vi "Untitled 1.vi"() -> ()   [LabVIEW 2017]
uses:
  <vilib>/Platform/TimedLoop/XDataNode/timing_clust.ctl
  <vilib>/Platform/TimedLoop/XDataNode/nitl_modes.ctl
  <vilib>/Platform/TimedLoop/XDataNode/wakeup.ctl
  <vilib>/platform/TimedLoop/XDataNode/XDataNode.xnode
  <vilib>/Platform/TimedLoop/XDataNode/XDNodeRunTimeDep.lvlib
panel:
  in  "Initialize integral 2":bool
  out "Analog2":dbl(knob) scale=0.0..5.0
  out "Waveform Chart 2":cluster{"Ref2":dbl, dbl}(graph)
  out "Pos2":dbl(knob) scale=0.0..360.0
  in  "Ref2":dbl(slide) scale=-720.0..720.0
  in  "stop":bool
  in  "Kd":dbl(slide) scale=0.0..10.0
  in  "Ki":dbl(slide) scale=0.0..10.0
  in  "Kp":dbl(slide) scale=0.0..10.0
  out "Analog1":dbl(knob) scale=0.0..5.0
  out "Waveform Chart":cluster{"Ref 1":dbl, dbl}(graph)
  in  "Initialize integral 1":bool
  in  "Ref 1":dbl(slide) scale=-720.0..720.0
  out "Pos 1":dbl(knob) scale=0.0..360.0
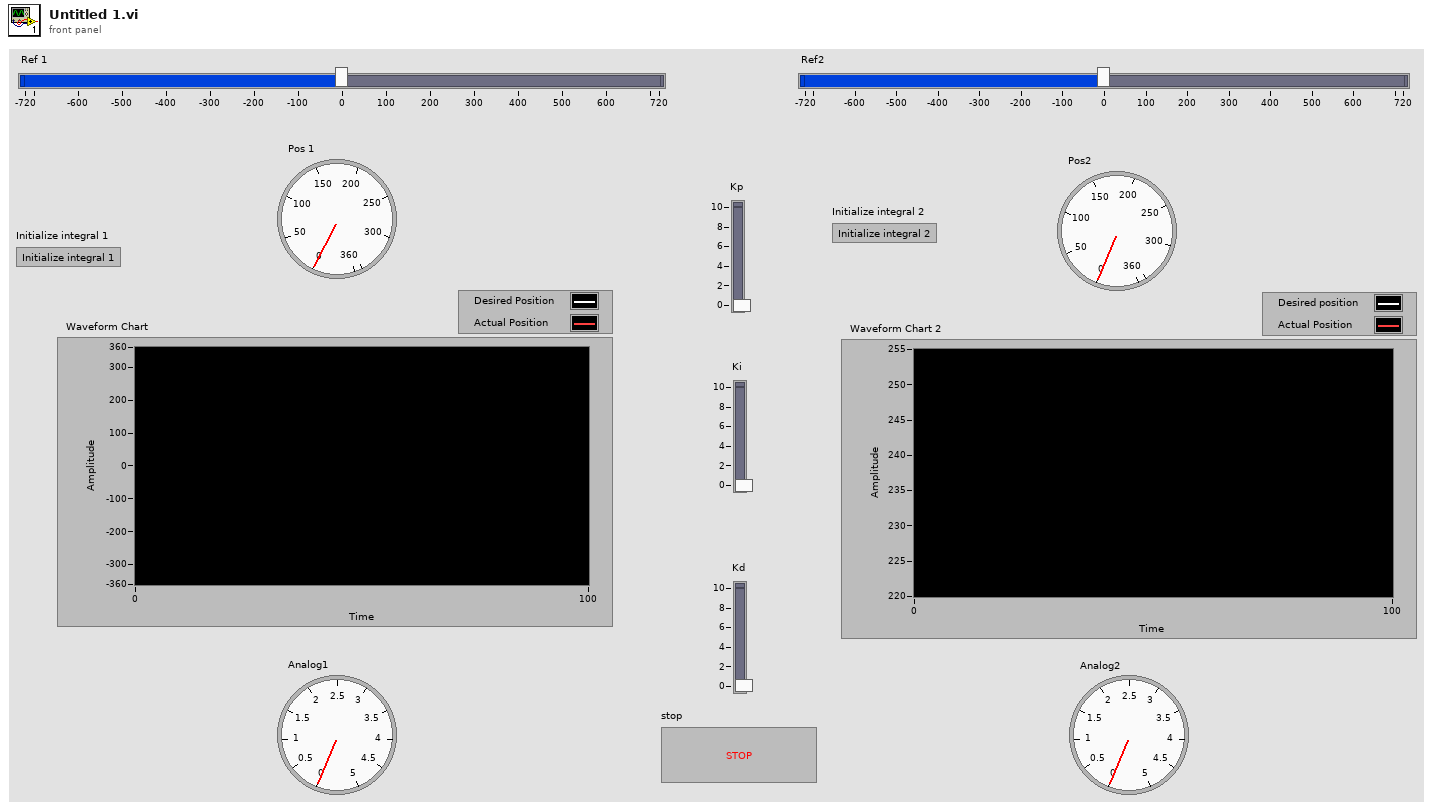
[diagram p1: front panel]
types:
  T1 = typedef "XDNodeRunTimeDep.lvlib/timing_clust.ctl" = cluster{"Expected End [f-1]":u64, "Actual End [f-1]":u64, "Finished Late? [f-1]":bool, "Expected End [i-1]":u64, "Actual End [i-1]":u64, "Finished Late? [i-1]":bool, "Expected Start [i]":u64, "Actual Start [i]":u64, "Expected Start [f]":u64, "Actual Start [f]":u64, "Source Name":string, "Structure Name":string, "Period":i64, "Deadline":i64, "Offset":i64, "Start":i64, "Priority":i32, "Timeout":i32, "Mode":T2, "Wakeup Reason":T3, "Error":errorcluster, "Source Type":string, "Secondary Source Type":string, "Global End Time":u64, "Global Start Time":u64, "Frame Duration":u64, "Iteration Duration":u64, "Assigned CPU":i32, "I/O Scan Engine Mode":u32}
  T2 = typedef "XDNodeRunTimeDep.lvlib/nitl_modes.ctl" = enum32{"No Change", "Process missed periods, maintain original phase", "Discard missed periods, maintain original phase", "Process missed periods, ignore original phase", "Discard missed periods, ignore original phase"}
  T3 = typedef "XDNodeRunTimeDep.lvlib/wakeup.ctl" = enum32{"Normal", "Aborted", "Asynchronous wakeup", "Timing source error", "Timed loop error", "Timeout"}
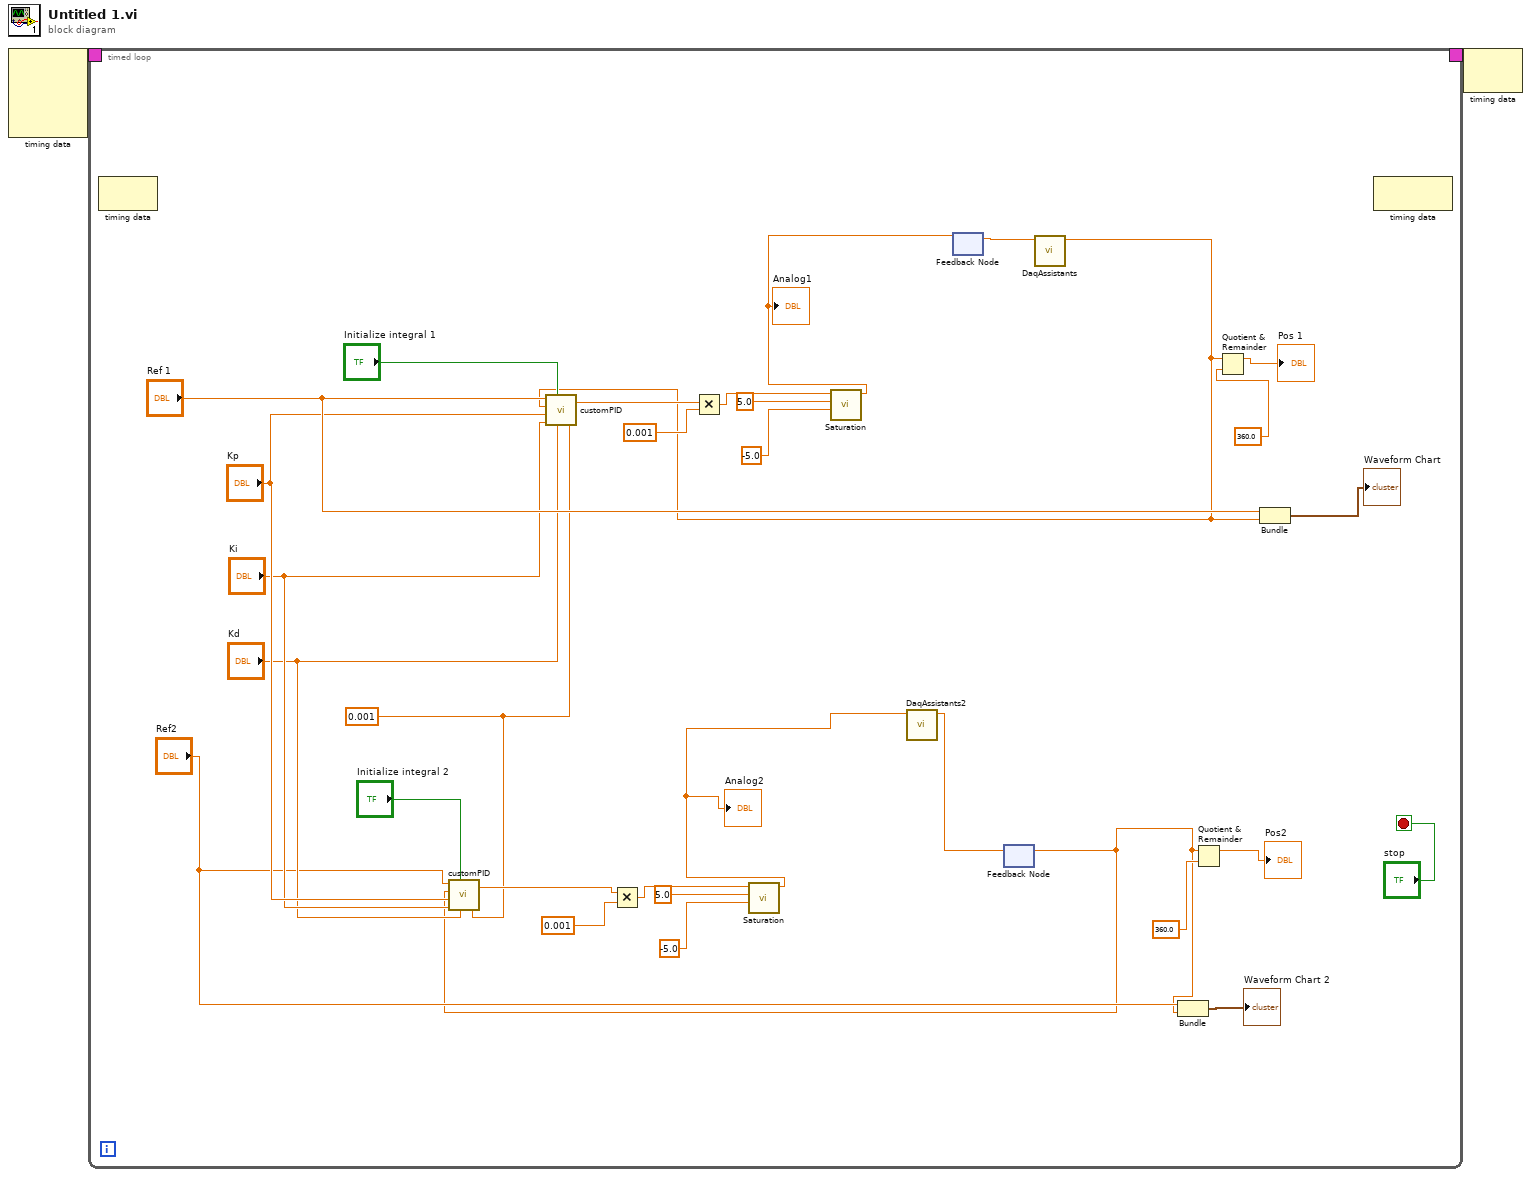
[diagram p0: block diagram]
diagram:
  n1 = node-c288() -> (w2:T1)  [unwired: 4 in]
  n2 = timed-loop {
    timing: w2 -> [_]
    timing-out: [_] -> w1
    stop <- "stop" stop-if-true
    w11 = 0.001
    n3 = node-c288() -> ()  [unwired: 1 in, 1 out]
    n4 = feedback #1() -> (w7:dbl)  [unwired: 1 in]
    n5 = feedback #2() -> (w3:dbl)  [unwired: 1 in]
    n6 = call "customPID.vi"("dt"=w11, "Kd"="Kd", "Initialize"="Initialize integral 2", "Ki"="Ki", "Kp"="Kp", "Measured"=w3, "Desired"="Ref2") -> ("Motor Input"=w15:dbl)
    n7 = Multiply(x=w15, y=0.001) -> (x*y=w22:dbl)
    n8 = call "Saturation.vi"("lower bound"=-5.0, "upper bound"=5.0, "input"=w22) -> ("output"=w5:dbl)  [unwired: 8 in]
    "Analog2" <- w5
    n9 = call "DaqAssistants2.vi"("output"=w5) -> ("Numeric"=w4:dbl)  [unwired: 10 in]
    n10 = feedback-in #2(w4) -> ()
    n11 = call "DaqAssistants.vi"("output"=w7) -> ("Numeric"=w6:dbl)  [unwired: 10 in]
    n12 = call "customPID.vi"("dt"=w11, "Kd"="Kd", "Initialize"="Initialize integral 1", "Ki"="Ki", "Kp"="Kp", "Measured"=w6, "Desired"="Ref 1") -> ("Motor Input"=w31:dbl)
    n13 = Multiply(x=w31, y=0.001) -> (x*y=w30:dbl)
    n14 = call "Saturation.vi"("lower bound"=-5.0, "upper bound"=5.0, "input"=w30) -> ("output"=w8:dbl)  [unwired: 8 in]
    "Analog1" <- w8
    n15 = feedback-in #1(w8) -> ()
    n16 = Bundle("Ref2"="Ref2", "Numeric"=w3) -> (→"Waveform Chart 2":cluster{"Ref2":dbl, "Numeric":dbl})  [unwired: 1 in]
    n17 = Quotient & Remainder(x=w3, y=360.0) -> (x-y*floor(x/y)=→"Pos2":dbl)  [unwired: 1 out]
    n18 = Quotient & Remainder(x=w6, y=360.0) -> (x-y*floor(x/y)=→"Pos 1":dbl)  [unwired: 1 out]
    n19 = Bundle("Ref 1"="Ref 1", "Numeric"=w6) -> (→"Waveform Chart":cluster{"Ref 1":dbl, "Numeric":dbl})  [unwired: 1 in]
    n20 = node-c288() -> ()  [unwired: 1 in, 1 out]
  }
  n21 = node-c288(w1) -> ()  [unwired: 1 out]
